vi "DriveStraight.vi"(10 "Drive Distance (in)":dbl) -> ()   [LabVIEW 2012]
uses:
  System Set Points and States.vi
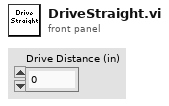
[diagram p1: front panel]
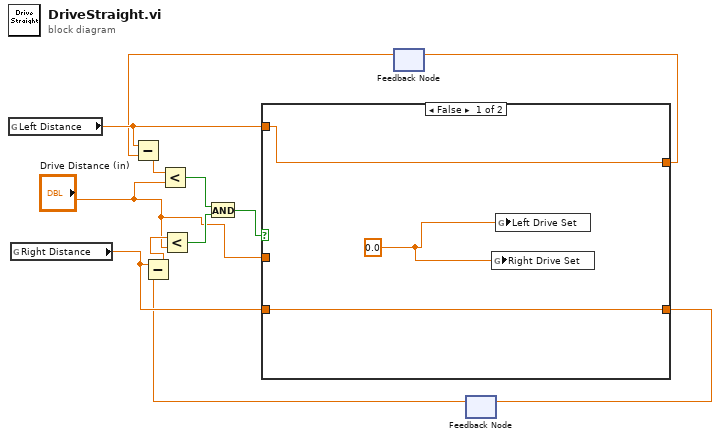
[diagram p0: block diagram]
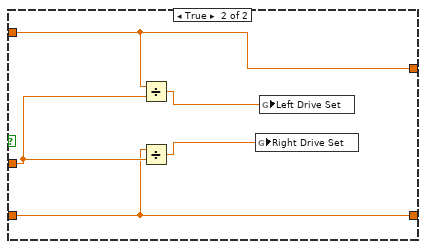
[diagram p2: hidden frame]
diagram:
  n1 = global read "System Set Points and States.vi" "Left Distance"() -> (w7:dbl)
  n2 = global read "System Set Points and States.vi" "Right Distance"() -> (w3:dbl)
  n3 = feedback #1() -> (w5:dbl)  [unwired: 1 in]
  n4 = Subtract(x=w7, y=w5) -> (x-y=w9:dbl)
  n5 = Less?(x=w9, y="Drive Distance (in)") -> (x < y?=w10:bool)
  n6 = feedback #2() -> (w2:dbl)  [unwired: 1 in]
  n7 = Subtract(x=w3, y=w2) -> (x-y=w8:dbl)
  n8 = Less?(x=w8, y="Drive Distance (in)") -> (x < y?=w11:bool)
  n9 = And(x=w10, y=w11) -> (x .and. y?=w12:bool)
  n10 = case shown="False" w12 {
    tunnel: [w15 w20] -> w6
    tunnel: w7 -> [w15 w20]
    tunnel: [w14 w18] -> w4
    tunnel: w3 -> [w14 w18]
    tunnel: "Drive Distance (in)" -> [_ w19]
    frame False {
      w13 = 0.0 ("Left Drive JS")
      n11 = global write "System Set Points and States.vi" "Right Drive Set"(w13) -> ()
      n12 = global write "System Set Points and States.vi" "Left Drive Set"(w13) -> ()
    }
    frame True {
      n13 = Divide(x=w20, y=w19) -> (x/y=w17:dbl)
      n14 = Divide(x=w18, y=w19) -> (x/y=w16:dbl)
      n15 = global write "System Set Points and States.vi" "Right Drive Set"(w16) -> ()
      n16 = global write "System Set Points and States.vi" "Left Drive Set"(w17) -> ()
    }
  }
  n17 = feedback-in #1(w6) -> ()
  n18 = feedback-in #2(w4) -> ()
